vi "Close Control.vi"(8 "error in (no error)":errorcluster, 11 "SingleStepTestV3 in":refnum<class "SingleStepTestV3.lvclass">) -> (0 "error out":errorcluster, 3 "SingleStepTestV3 out":refnum<class "SingleStepTestV3.lvclass">)   [LabVIEW 2016, in "SingleStepTestV3.lvlib" / "SingleStepTestV3.lvclass"]
doc: "The <b>Close Control VI</b> is a dynamic dispatch VI that must be used in the cleanup of portion of the calling code before ending.\n\nIt should be overwritten if the QControl Class needs to do any uninitialization or closing of references.\n\nIf overwritten, the <b>Call Parent Method</b> must be called in order to cleanup the control reference, close running <b>Event Handler VI</b> (if there is one), and release the State Data DVR (if there is one).\n<b> </b> <b> </b>\n©2016 Q Software Innovations, LLC (QSI)\nwritten by Quentin Alldredge\nproduced in LabVIEW 2015\n\nsupport@qsoftwareinnovations.com\nwww.qsoftwareinnovations.com\n\nAll rights reserved.\n\nRedistribution and use in source and binary forms, with or without modification, are permitted provided that the following conditions are met:\n\n * Redistributions of source code must retain the above copyright notice, this list of conditions and the following disclaimer.\n * Redistributions in binary form must reproduce the above copyright notice, this list of conditions and the following disclaimer in the documentation and/or other materials provided with the distribution.\n * Neither the name of Q Software Innovations, LLC. nor the names of its contributors may be used to endorse or promote products derived from this software without specific prior written permission.\n\nTHIS SOFTWARE IS PROVIDED BY THE COPYRIGHT HOLDERS AND CONTRIBUTORS \"AS IS\" AND ANY EXPRESS OR IMPLIED WARRANTIES, INCLUDING, BUT NOT LIMITED TO, THE IMPLIED WARRANTIES OF MERCHANTABILITY AND FITNESS FOR A PARTICULAR PURPOSE ARE DISCLAIMED. IN NO EVENT SHALL THE COPYRIGHT OWNER OR CONTRIBUTORS BE LIABLE FOR ANY DIRECT, INDIRECT, INCIDENTAL, SPECIAL, EXEMPLARY, OR CONSEQUENTIAL DAMAGES (INCLUDING, BUT NOT LIMITED TO, PROCUREMENT OF SUBSTITUTE GOODS OR SERVICES; LOSS OF USE, DATA, OR PROFITS; OR BUSINESS INTERRUPTION) HOWEVER CAUSED AND ON ANY THEORY OF LIABILITY, WHETHER IN CONTRACT, STRICT LIABILITY, OR TORT (INCLUDING NEGLIGENCE OR OTHERWISE) ARISING IN ANY WAY OUT OF THE USE OF THIS SOFTWARE, EVEN IF ADVISED OF THE POSSIBILITY OF SUCH DAMAGE."
uses:
  SingleStepTestV3.lvclass
  <vilib>/QSI/QControls/QControl Classes/Cluster/Cluster.lvclass
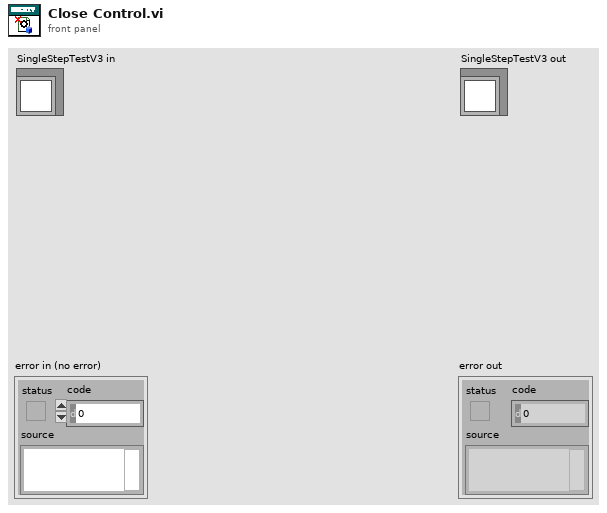
[diagram p1: front panel]
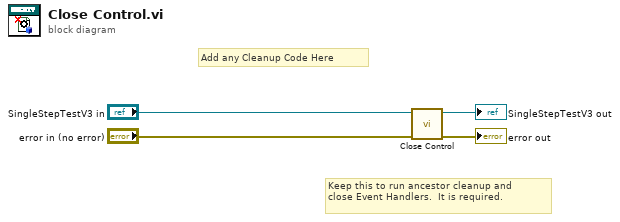
[diagram p0: block diagram]
diagram:
  # "Keep this to run ancestor cleanup and\nclose Event Handlers.  It is required."
  # "Add any Cleanup Code Here"
  n1 = call-parent "Close Control.vi"("error in (no error)"="error in (no error)", "Control in"="SingleStepTestV3 in") -> ("error out"=→"error out":errorcluster, "Control out"=→"SingleStepTestV3 out":refnum<class "SingleStepTestV3.lvclass">)  [unwired: 8 in]
